vi "Save_data_txt.vi"(8 "error in (no error)":errorcluster, 10 "Grafica":waveform(dbl)(graph), 11 "Logging_txt in":refnum<class "Logging_txt.lvclass">) -> (0 "error out":errorcluster, 3 "Logging_txt out":refnum<class "Logging_txt.lvclass">)   [LabVIEW 2019, in "Logging_txt.lvlib" / "Logging_txt.lvclass"]
uses:
  Logging_txt.lvclass
  Logging_txt.lvclass/Logging_txt.ctl
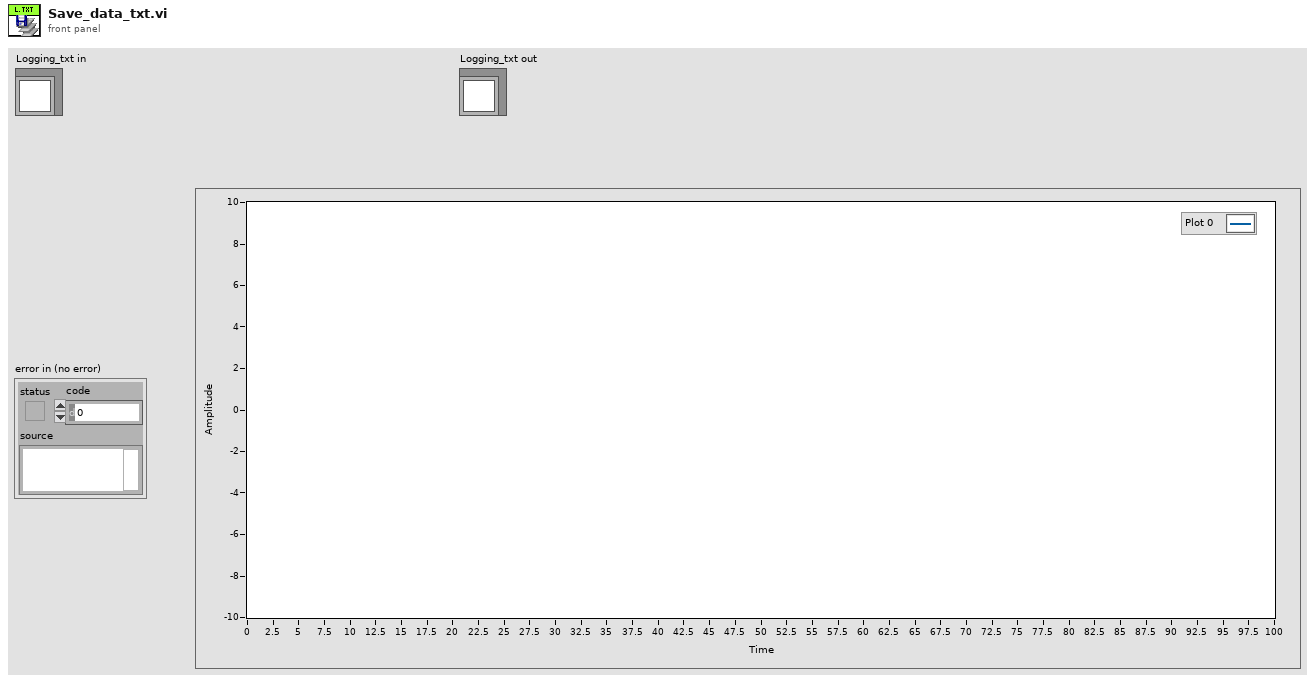
[diagram p1: front panel]
types:
  T1 = enum16{"open", "replace", "create", "open or create", "replace or create", "replace or create with confirmation"}
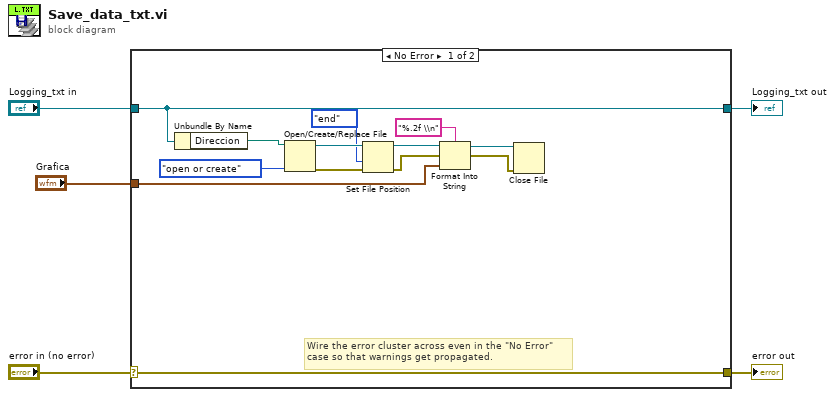
[diagram p0: block diagram]
diagram:
  n1 = case shown="No Error" "error in (no error)" {
    selector: "error in (no error)" -> [w18 w20]
    tunnel: [w18 w20] -> w4
    tunnel: [w17 w19] -> w2
    tunnel: "Logging_txt in" -> [w17 w19]
    tunnel: "Grafica" -> [w7 _]
    frame No Error {
      # "Wire the error cluster across even in the \"No Error\"\ncase so that warnings get propagated."
      n2 = Unbundle By Name(w17) -> ("Direccion"=w16:path)
      n3 = Open/Create/Replace File(file path (use dialog)=w16, operation (0:open)=T1."open or create") -> (refnum out=w14:refnum<file>, error out=w12:errorcluster)  [unwired: 4 in, 1 out]
      n4 = Set File Position(refnum=w14, from (0:start)=enum16{"start", "end", "current"}."end", error in=w12) -> (refnum out=w13:refnum<file>, error out=w11:errorcluster)  [unwired: 1 in]
      n5 = Format Into String(format string="%.2f \\n", initial string=w13, error in=w11, w7) -> (resulting string=w10:refnum<file>, error out=w9:errorcluster)
      n6 = Close File(refnum=w10, error in=w9) -> ()  [unwired: 2 out]
    }
    frame Error {
    }
  }
  "error out" <- w4
  "Logging_txt out" <- w2
